vi "Get file and folder data.vi"(5 "Sorted string path":string[](array[string]), 11 "Error in":errorcluster) -> (4 "file/folder data":string[][](array[string]), 15 "Error out":errorcluster)   [LabVIEW 2020, in "Custom Sort Function.lvlib"]
uses:
  Libraries/Custom Sort Function.lvlib
panel:
  # "Get file size and folder data"
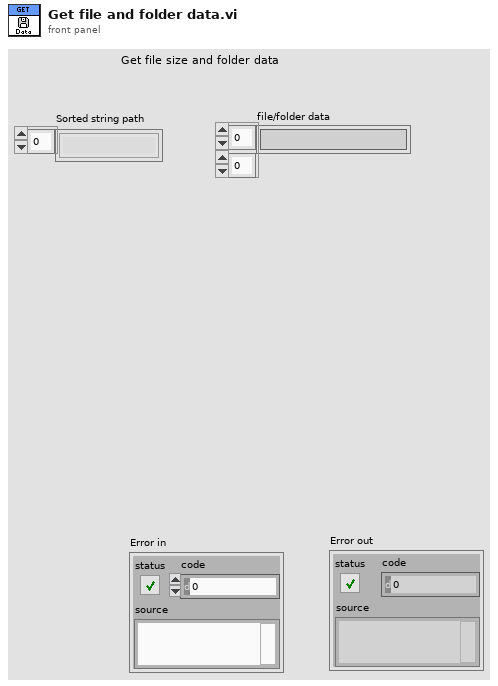
[diagram p1: front panel]
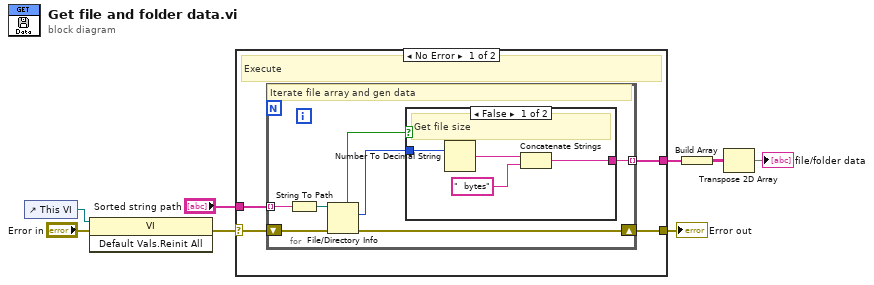
[diagram p0: block diagram]
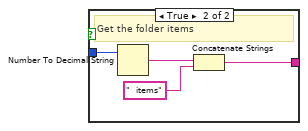
[diagram p2: hidden frame]
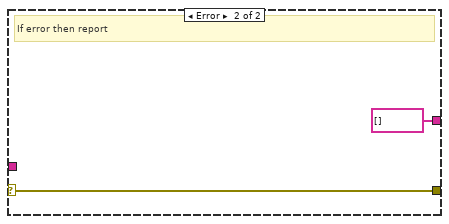
[diagram p3: hidden frame]
diagram:
  n1 = control-ref of="This VI"() -> (w3:refnum<vi>)
  n2 = invoke class="VI" method="Default Vals.Reinit All"(reference=w3, error in="Error in") -> (error out=w2:errorcluster)  [unwired: 1 in, 2 out]
  n3 = case shown="No Error" w2 {
    selector: w2 -> [w12 w29]
    tunnel: [w11 w29] -> w8
    tunnel: [w10 string[] []] -> w6
    tunnel: "Sorted string path" -> [w9 _]
    frame No Error {
      # "Execute"
      n4 = for {
        tunnel: [w15] -> w10 mode=indexing
        shift-right: [w18] -> w11
        shift-left: w12 -> [w19]
        tunnel: w9 -> [w13] mode=indexing
        # "Iterate file array and gen data"
        n5 = String To Path(string=w13) -> (path=w14:path)
        n6 = File/Directory Info(path=w14, error in=w19) -> (directory=w17:bool, size=w16:i64, error out=w18:errorcluster)  [unwired: 4 out]
        n7 = case shown="False" w17 {
          tunnel: w16 -> [w21 w27]
          tunnel: [w20 w24] -> w15
          frame False {
            # "Get file size"
            n8 = Number To Decimal String(number=w21) -> (decimal integer string=w23:string)  [unwired: 1 in]
            n9 = Concatenate Strings(w23, "  bytes" ("string")) -> (w20:string)
          }
          frame True {
            # "Get the folder items"
            n10 = Number To Decimal String(number=w27) -> (decimal integer string=w26:string)  [unwired: 1 in]
            n11 = Concatenate Strings(w26, "  items" ("string")) -> (w24:string)
          }
        }
      }
    }
    frame Error {
      # "If error then report"
    }
  }
  "Error out" <- w8
  n12 = Build Array(w6) -> (w5:string[][])
  n13 = Transpose 2D Array(2D array=w5) -> (transposed array=→"file/folder data":string[][])
